vi "Render.vi"(7 "Data":refnum<class "Datum.lvclass">, 8 "Error In":errorcluster, 10 "Abstract Syntax Tree":refnum<class "Root.lvclass">, 11 "Compiler In":refnum<class "Compiler.lvclass">) -> (0 "Error Out":errorcluster, 3 "Compiler Out":refnum<class "Compiler.lvclass">)   [LabVIEW 2018, in "Toolkit.lvlib" / "Compiler.lvclass"]
uses:
  Compiler.lvclass
  Nodes/Root/Root.lvclass
  Data/Datum/Datum.lvclass
  Compiler.lvclass/Compiler.ctl
  Renderer/Renderer.lvclass
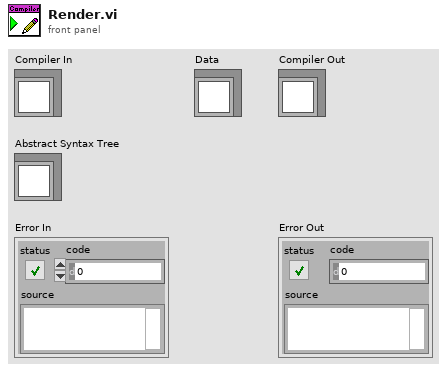
[diagram p1: front panel]
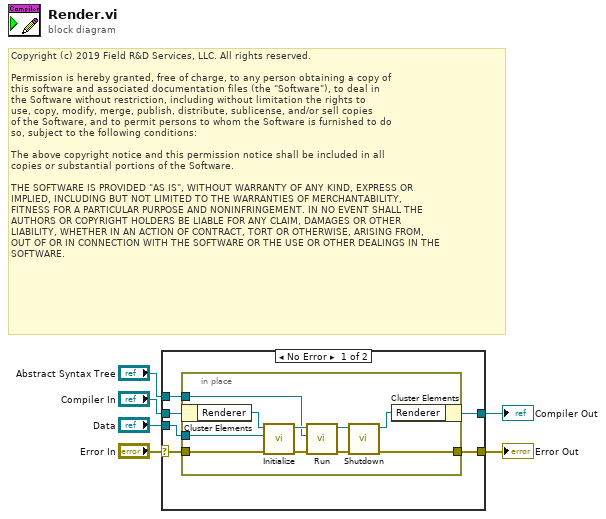
[diagram p0: block diagram]
diagram:
  # "Copyright (c) 2019 Field R&D Services, LLC. All rights reserved.\n\nPermission is hereby granted, free of charge, to any person obtaining a copy of\nthis software and associated documentation files (the \"Software\"), to deal in\nthe Software without restriction, including without limitation the rights to\nuse, copy, modify, merge, publish, distribute, sublicense, and/or sell copies\nof the Software, and to permit persons to whom the Software is furnished to do\nso, subject to the following conditions:\n\nThe above copyright notice and this permission notice shall be included in all\ncopies or substantial portions of the Software.\n\nTHE SOFTWARE IS PROVIDED \"AS IS\", WITHOUT WARRANTY OF ANY KIND, EXPRESS OR\nIMPLIED, INCLUDING BUT NOT LIMITED TO THE WARRANTIES OF MERCHANTABILITY,\nFITNESS FOR A PARTICULAR PURPOSE AND NONINFRINGEMENT. IN NO EVENT SHALL THE\nAUTHORS OR COPYRIGHT HOLDERS BE LIABLE FOR ANY CLAIM, DAMAGES OR OTHER\nLIABILITY, WHETHER IN AN ACTION OF CONTRACT, TORT OR OTHERWISE, ARISING FROM,\nOUT OF OR IN CONNECTION WITH THE SOFTWARE OR THE USE OR OTHER DEALINGS IN THE\nSOFTWARE."
  n1 = case shown="No Error" "Error In" {
    selector: "Error In" -> [w11 w24]
    tunnel: [w9 w24] -> w5
    tunnel: "Compiler In" -> [w12 w23]
    tunnel: [w10 w23] -> w3
    tunnel: "Abstract Syntax Tree" -> [w8 _]
    tunnel: "Data" -> [w7 _]
    frame No Error {
      n2 = in-place {
        in-place-border: w11 -> [w21]
        in-place-border: [w22] -> w9
        in-place-border: w8 -> [w14]
        in-place-border: w7 -> [w13]
        n3 = in-place-cluster #1(w12) -> ("Renderer"=w20:refnum<class "Renderer.lvclass">)
        n4 = call-dynamic "Initialize.vi"("Error In"=w21, "Data"=w13, "Renderer In"=w20) -> ("Error Out"=w16:errorcluster, "Renderer Out"=w18:refnum<class "Renderer.lvclass">)  [unwired: 7 in]
        n5 = call-dynamic "Run.vi"("Error In"=w16, "Abstract Syntax Tree"=w14, "Renderer In"=w18) -> ("Error Out"=w15:errorcluster, "Renderer Out"=w17:refnum<class "Renderer.lvclass">)  [unwired: 7 in]
        n6 = call-dynamic "Shutdown.vi"("Error In"=w15, "Renderer In"=w17) -> ("Error Out"=w22:errorcluster, "Renderer Out"=w19:refnum<class "Renderer.lvclass">)  [unwired: 7 in, 1 out]
        n7 = in-place-cluster #1("Renderer"=w19) -> (w10:refnum<class "Compiler.lvclass">)
      }
    }
    frame Error {
    }
  }
  "Error Out" <- w5
  "Compiler Out" <- w3
